vi "PolyScopeVersion.vi"(0 "DashboardServer in":refnum<class "Dashboard Server.lvclass">, 5 "error in (no error)":errorcluster) -> (14 "DashboardServer out":refnum<class "Dashboard Server.lvclass">, 16 "PolyScopeVersion":string, 19 "error out":errorcluster)   [LabVIEW 2016, in "Dashboard Server.lvclass"]
uses:
  Dashboard Server.lvclass
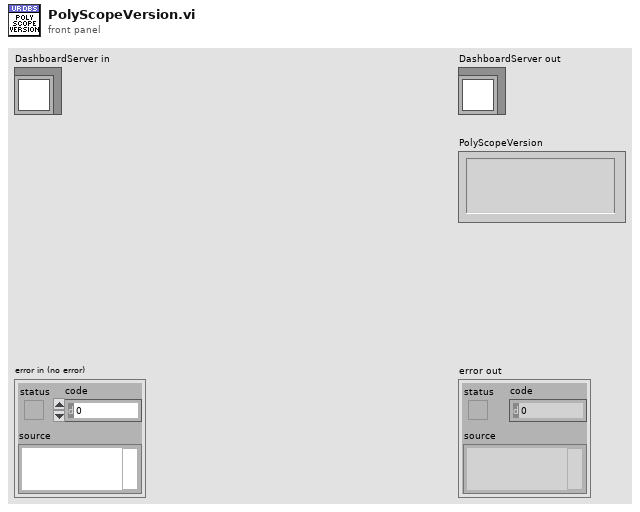
[diagram p1: front panel]
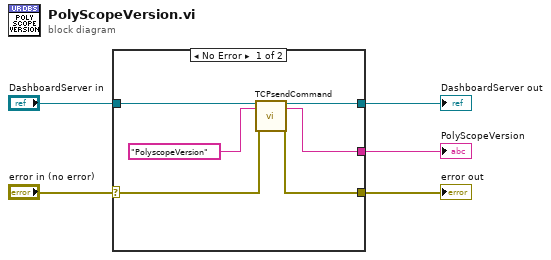
[diagram p0: block diagram]
diagram:
  n1 = case shown="No Error" "error in (no error)" {
    selector: "error in (no error)" -> [w9 w13]
    tunnel: [w8 w13] -> w4
    tunnel: [w10 w12] -> w2
    tunnel: "DashboardServer in" -> [w11 w12]
    tunnel: [w6 _] -> w1
    frame No Error {
      n2 = call-dynamic "TCPsendCommand.vi"("DashboardServer in"=w11, "command"="PolyscopeVersion", "error in (no error)"=w9) -> ("DashboardServer out"=w10:refnum<class "Dashboard Server.lvclass">, "returnStatus"=w6:string, "error out"=w8:errorcluster)  [unwired: 13 in, 1 out]
    }
    frame Error {
    }
  }
  "error out" <- w4
  "DashboardServer out" <- w2
  "PolyScopeVersion" <- w1
